vi "Day11-03_TCP 통신.vi"() -> ()   [LabVIEW 2021]
panel:
  in  "QUIT":bool
  in  "PLAY":bool
  in  "INIT":bool
  out "데이터 출력":string
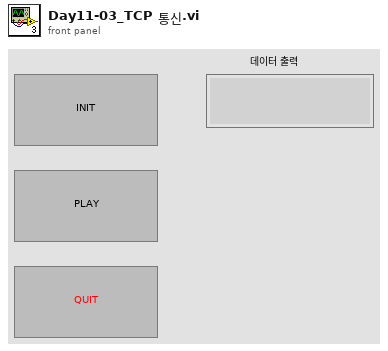
[diagram p1: front panel]
types:
  T1 = enum16{"Standard", "Buffered", "CRLF", "Immediate"}
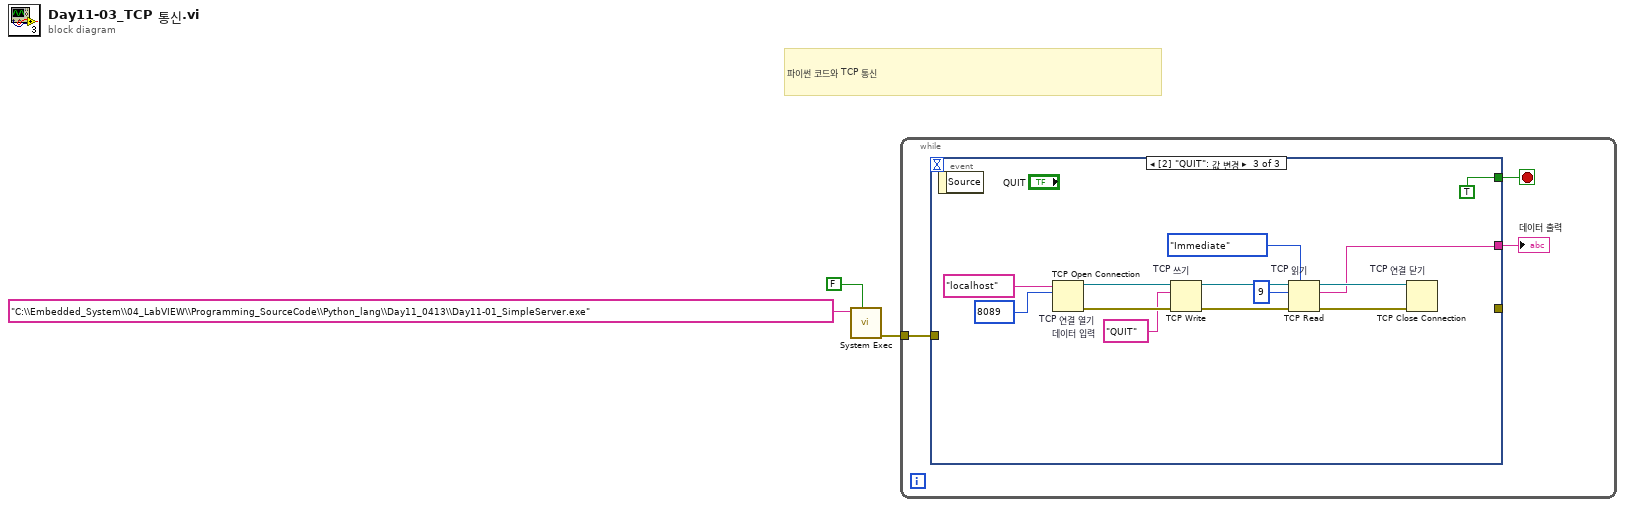
[diagram p0: block diagram]
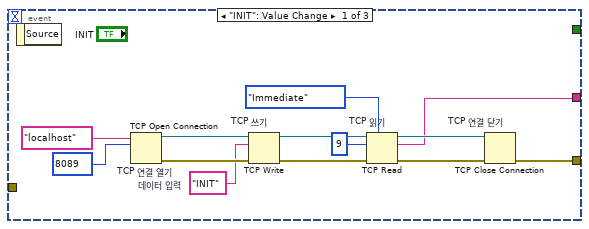
[diagram p2: hidden frame]
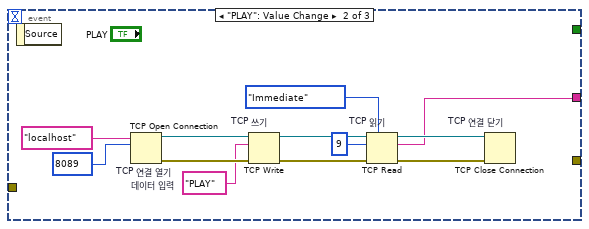
[diagram p3: hidden frame]
diagram:
  # "파이썬 코드와 TCP 통신"
  n1 = call <vilib>:"System Exec.vi"("wait until completion? (T)"=FALSE, "command line"="C:\\Embedded_System\\04_LabVIEW\\Programming_SourceCode\\Python_lang\\Day11_0413\\Day11-01_SimpleServer.exe") -> ("error out"=w1:errorcluster)  [unwired: 6 in, 3 out]
  n2 = while {
    tunnel: w1 -> [w4]
    stop <- w5 stop-if-true
    n3 = event shown="[2] \"QUIT\": 값 변경" {
      selector: _ -> [_ _ _]
      dyn-events: _ -> [_ _ _]
      timeout: _ -> [_ _ _]
      tunnel: [w8 w20 w33] -> w6
      tunnel: [_ _ TRUE] -> w5
      tunnel: [w7 _ _] -> _
      tunnel: w4 -> [_ _ _]
      event "INIT": Value Change {
        w11 = "INIT"  # 데이터 입력
        n4 = event-data() -> ()  [unwired: 1 in, 1 out]
        n5 = TCP Open Connection "TCP 연결 열기"(address="localhost" ("주소"), remote port or service name=u16 8089 ("원격 포트 또는 서비스 이름")) -> (connection ID=w17:refnum<k5>, error out=w16:errorcluster)  [unwired: 3 in]
        n6 = TCP Write "TCP 쓰기"(connection ID=w17, data in=w11, error in (no error)=w16) -> (connection ID out=w15:refnum<k5>, error out=w14:errorcluster)  [unwired: 1 in, 1 out]
        n7 = TCP Read "TCP 읽기"(connection ID=w15, bytes to read=9 ("읽을 바이트"), error in (no error)=w14, 7:T1."Immediate" ("모드(standard)")) -> (connection ID out=w13:refnum<k5>, data out=w8:string, error out=w12:errorcluster)  [unwired: 1 in]
        n8 = TCP Close Connection "TCP 연결 닫기"(connection ID=w13, error in (no error)=w12) -> (error out=w7:errorcluster)  [unwired: 1 in, 1 out]
      }
      event "PLAY": Value Change {
        w23 = "PLAY"  # 데이터 입력
        n9 = event-data() -> ()  [unwired: 1 in, 1 out]
        n10 = TCP Open Connection "TCP 연결 열기"(address="localhost" ("주소"), remote port or service name=u16 8089 ("원격 포트 또는 서비스 이름")) -> (connection ID=w29:refnum<k5>, error out=w28:errorcluster)  [unwired: 3 in]
        n11 = TCP Write "TCP 쓰기"(connection ID=w29, data in=w23, error in (no error)=w28) -> (connection ID out=w27:refnum<k5>, error out=w26:errorcluster)  [unwired: 1 in, 1 out]
        n12 = TCP Read "TCP 읽기"(connection ID=w27, bytes to read=9 ("읽을 바이트"), error in (no error)=w26, 7:T1."Immediate" ("모드(standard)")) -> (connection ID out=w25:refnum<k5>, data out=w20:string, error out=w24:errorcluster)  [unwired: 1 in]
        n13 = TCP Close Connection "TCP 연결 닫기"(connection ID=w25, error in (no error)=w24) -> ()  [unwired: 1 in, 2 out]
      }
      event "QUIT": Value Change {
        w36 = "QUIT"  # 데이터 입력
        n14 = event-data() -> ()  [unwired: 1 in, 1 out]
        n15 = TCP Open Connection "TCP 연결 열기"(address="localhost" ("주소"), remote port or service name=u16 8089 ("원격 포트 또는 서비스 이름")) -> (connection ID=w42:refnum<k5>, error out=w41:errorcluster)  [unwired: 3 in]
        n16 = TCP Write "TCP 쓰기"(connection ID=w42, data in=w36, error in (no error)=w41) -> (connection ID out=w40:refnum<k5>, error out=w39:errorcluster)  [unwired: 1 in, 1 out]
        n17 = TCP Read "TCP 읽기"(connection ID=w40, bytes to read=9 ("읽을 바이트"), error in (no error)=w39, 7:T1."Immediate" ("모드(standard)")) -> (connection ID out=w38:refnum<k5>, data out=w33:string, error out=w37:errorcluster)  [unwired: 1 in]
        n18 = TCP Close Connection "TCP 연결 닫기"(connection ID=w38, error in (no error)=w37) -> ()  [unwired: 1 in, 2 out]
      }
    }
    "데이터 출력" <- w6
  }
